vi "Database Command Set Parameter Value.vi"(8 "error in (no error)":errorcluster caption="错误输入（无错误）", 9 "Value":variant, 10 "Index":i32, 11 "Database Command 输入":refnum<class "Database Command.lvclass"> caption="DNL_LabVIEW Object in") -> (0 "error out":errorcluster caption="错误输出", 3 "Database Command 输出":refnum<class "Database Command.lvclass"> caption="DNL_LabVIEW Object out")   [LabVIEW 2011, in "Database Command.lvclass"]
uses:
  Database Command.lvclass
  Database Command.lvclass/Database Command.ctl
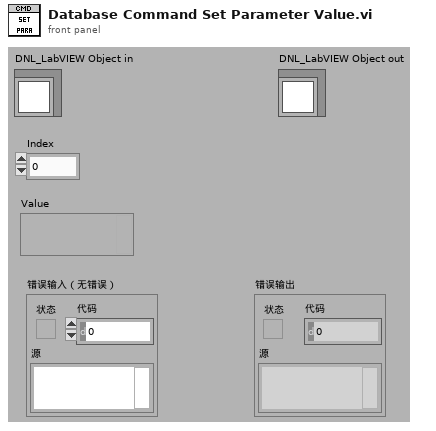
[diagram p1: front panel]
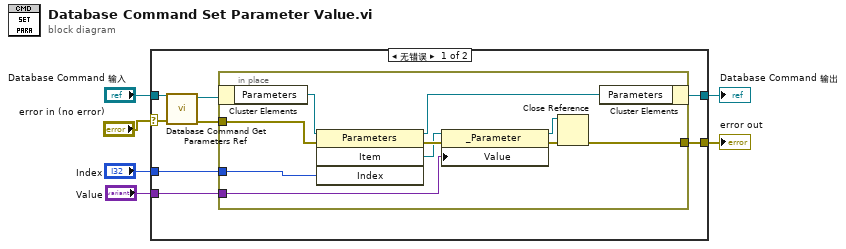
[diagram p0: block diagram]
diagram:
  n1 = case shown="无错误" "error in (no error)" {
    selector: "error in (no error)" -> [w8 w26]
    tunnel: [w11 w26] -> w5
    tunnel: [w14 w25] -> w3
    tunnel: "Database Command 输入" -> [w10 w25]
    tunnel: "Index" -> [w13 _]
    tunnel: "Value" -> [w12 _]
    frame No Error {
      n2 = call "Database Command Get Parameters Ref.vi"("error in (no error)"=w8, "Database Command 输入"=w10) -> ("error out"=w7:errorcluster, "Database Command 输出"=w9:refnum<class "Database Command.lvclass">)  [unwired: 8 in]
      n3 = in-place {
        in-place-border: w13 -> [w20]
        in-place-border: w12 -> [w15]
        in-place-border: [w17] -> w11
        in-place-border: w7 -> [w16]
        n4 = in-place-cluster #1(w9) -> ("Parameters"=w24:refnum<k7>)
        n5 = invoke class="Parameters" method="Item"(reference=w24, error in=w16, "Index"=w20) -> (reference out=w23:refnum<k7>, error out=w22:errorcluster, "Item"=w21:refnum<k7>)  [unwired: 1 in, 1 out]
        n6 = property class="_Parameter"(reference=w21, error in=w22, "Value"=w15) -> (reference out=w19:refnum<k7>, error out=w18:errorcluster)
        n7 = Close Reference(reference=w19, error in (no error)=w18) -> (error out=w17:errorcluster)
        n8 = in-place-cluster #1("Parameters"=w23) -> (w14:refnum<class "Database Command.lvclass">)
      }
    }
    frame Error {
    }
  }
  "error out" <- w5
  "Database Command 输出" <- w3
